vi "AdminPanel.vi"() -> ()   [LabVIEW 2021]
uses:
  Controls/Enum.ctl
  Controls/MySQL Credential Control.ctl
panel:
  in  "input 1":string
  out "data":variant[][](array[variant])
  in  "Add":bool
  out "error out":errorcluster
  in  "error in (no error)":errorcluster
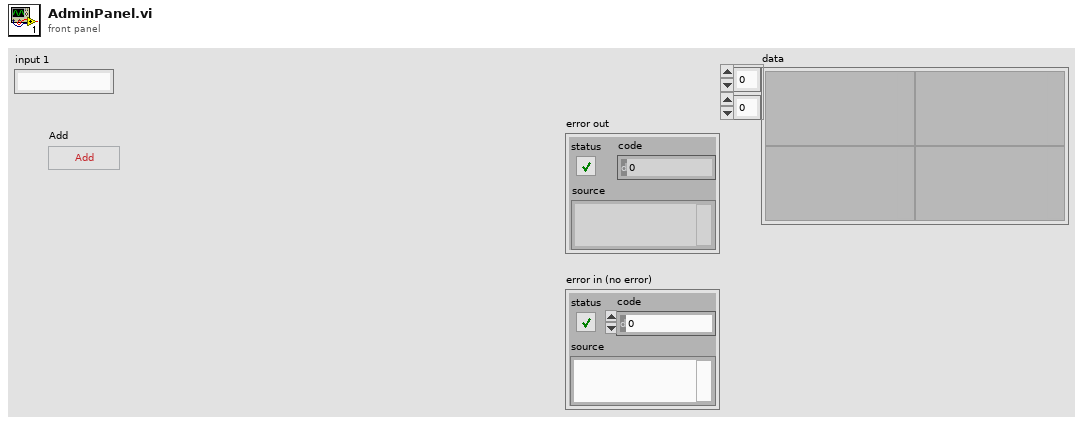
[diagram p1: front panel]
types:
  T1 = typedef "Enum.ctl" = enum16{"init", "Execute Query", "Close"}
  T2 = typedef "MySQL Credential Control.ctl" = cluster{"Server":string, " User ID":string, "Password":string}
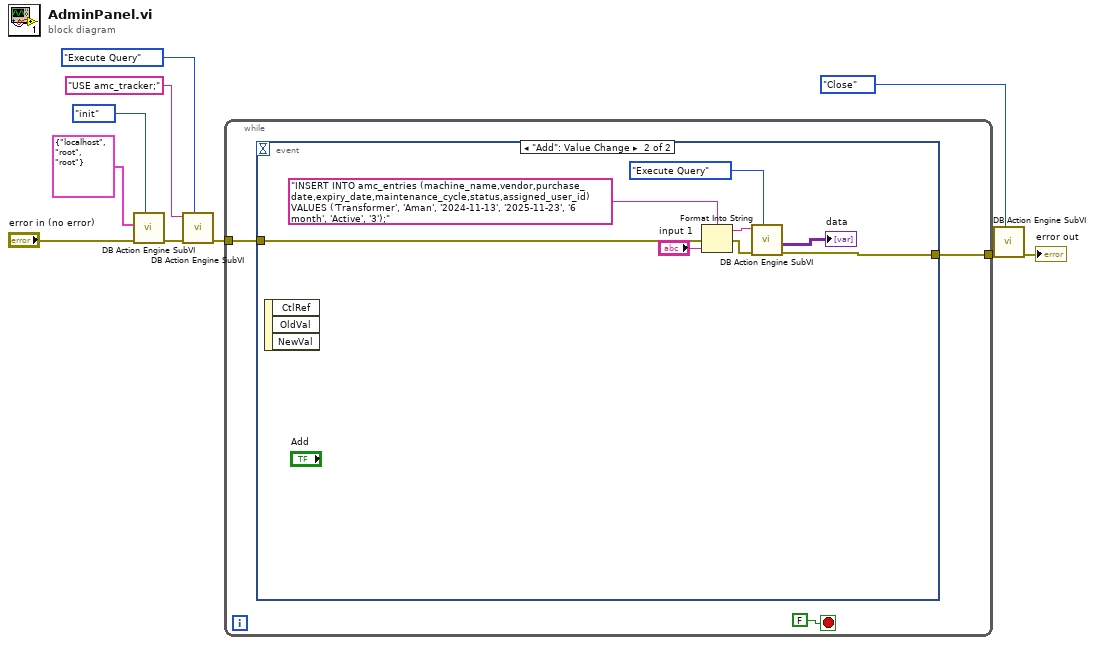
[diagram p0: block diagram]
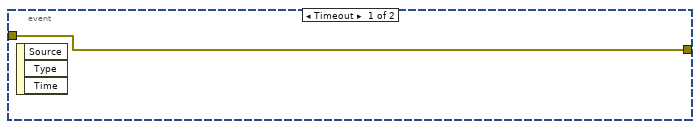
[diagram p2: hidden frame]
diagram:
  n1 = call "DB Action Engine SubVI.vi"("Cmd"=Enum."init", "error in (no error)"="error in (no error)", "MySQL Credentials"=T2 {"Server"="localhost", " User ID"="root", "Password"="root"}) -> ("error out"=w6:errorcluster)  [unwired: 6 in, 2 out]
  n2 = call "DB Action Engine SubVI.vi"("Cmd"=Enum."Execute Query", "error in (no error)"=w6, "Query String"="USE amc_tracker;") -> ("error out"=w4:errorcluster)  [unwired: 6 in, 2 out]
  n3 = while {
    tunnel: w4 -> [w13]
    tunnel: [w12] -> w3
    stop <- FALSE stop-if-true
    n4 = event shown="[1] \"Add\": Value Change" {
      selector: _ -> [_ _]
      dyn-events: _ -> [_ _]
      timeout: _ -> [_ _]
      tunnel: w13 -> [w14 w22]
      tunnel: [w14 w19] -> w12
      event Timeout {
        n5 = event-data() -> ()  [unwired: 1 in, 3 out]
      }
      event "Add": Value Change {
        n6 = event-data() -> ()  [unwired: 1 in, 3 out]
        n7 = Format Into String(format string="INSERT INTO amc_entries (machine_name,vendor,purchase_date,expiry_date,maintenance_cycle,status,assigned_user_id) VALUES ('Transformer', 'Aman', '2024-11-13', '2025-11-23', '6 month', 'Active', '3');", error in=w22, "input 1") -> (resulting string=w20:string, error out=w17:errorcluster)  [unwired: 1 in]
        n8 = call "DB Action Engine SubVI.vi"("Cmd"=Enum."Execute Query", "error in (no error)"=w17, "Query String"=w20) -> ("error out"=w19:errorcluster, "data"=→"data":variant[][])  [unwired: 6 in, 1 out]
      }
    }
  }
  n9 = call "DB Action Engine SubVI.vi"("Cmd"=Enum."Close", "error in (no error)"=w3) -> ("error out"=→"error out":errorcluster)  [unwired: 7 in, 2 out]
